vi "GetAlarms.vi"(0 "reference in":refnum<class "Stand.lvclass">, 11 "error in (no error)":errorcluster) -> (4 "reference out":refnum<class "Stand.lvclass">, 6 "Alarm":bool, 8 "Warning":bool, 15 "error out":errorcluster)   [LabVIEW 2019, in "Stand.lvclass"]
uses:
  Stand.lvclass
  Stand.lvclass/Stand.ctl
  PM_Group_class/PM_Group.lvclass
  C:/Users/ANENKOV_V1/Desktop/src/Proccess_class/Proccess.lvclass
  NeedleValve_class/NeedleValve.lvclass
  AI_class/AI.lvclass
  DI_class/DI.lvclass
  Valve_2DO_2DI_class/Valve_2DO_2DI.lvclass
  DA_class/DA.lvclass
  Proccess_class/Proccess.lvclass
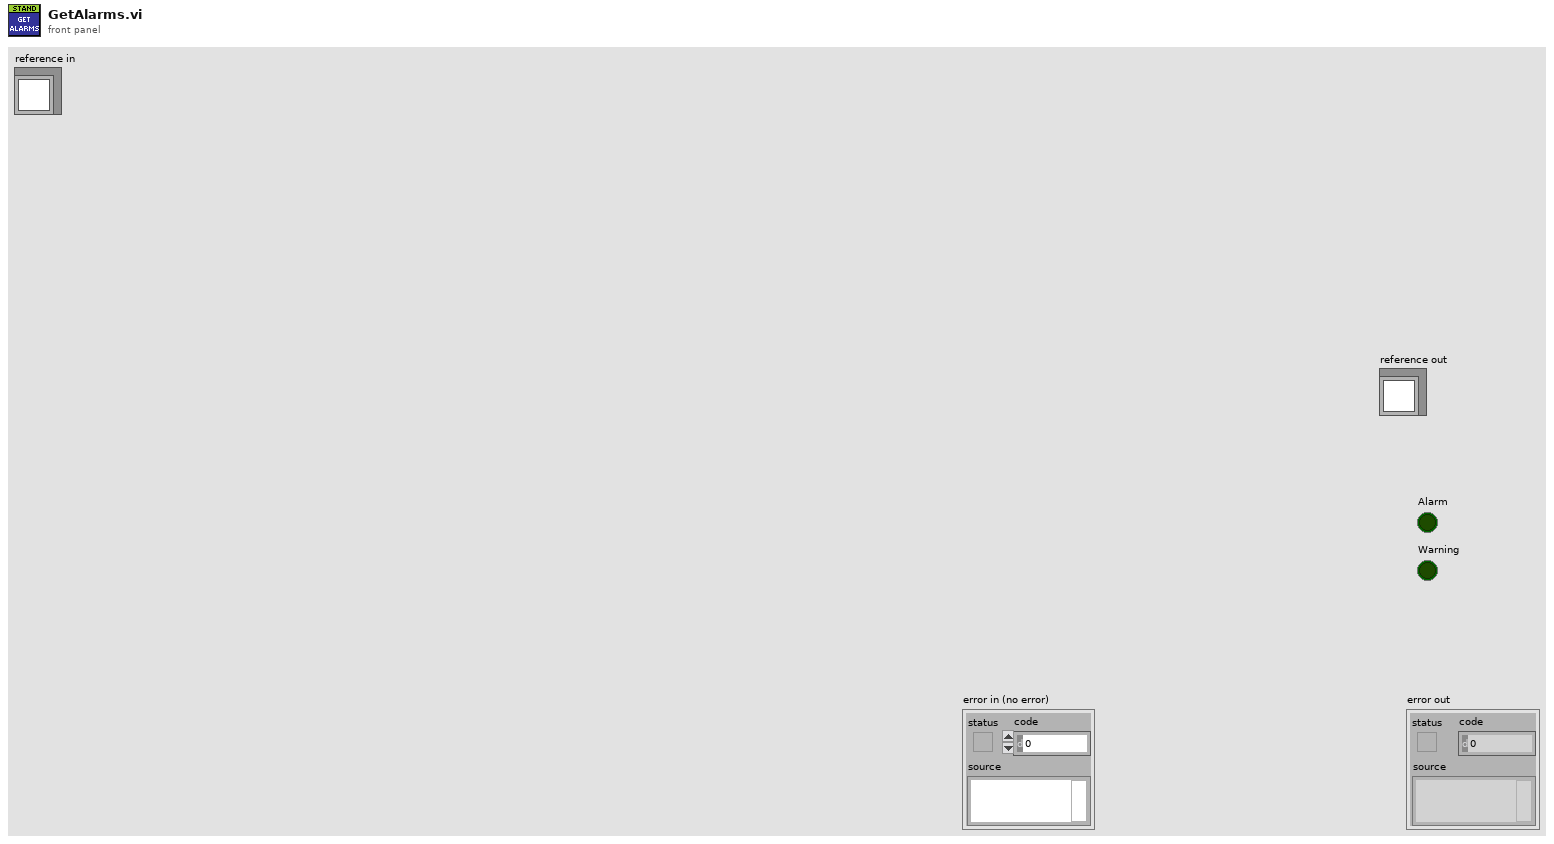
[diagram p1: front panel]
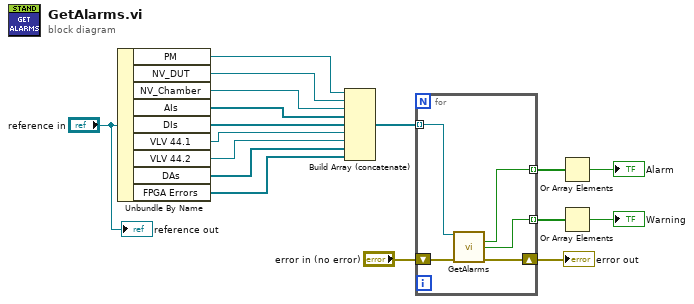
[diagram p0: block diagram]
diagram:
  n1 = Unbundle By Name("reference in") -> ("PM"=w9:refnum<class "PM_Group.lvclass">, "NV_DUT"=w8:refnum<class "NeedleValve.lvclass">, "NV_Chamber"=w7:refnum<class "NeedleValve.lvclass">, "AIs"=w6:refnum<class "AI.lvclass">[], "DIs"=w5:refnum<class "DI.lvclass">[], "VLV 44.1"=w4:refnum<class "Valve_2DO_2DI.lvclass">, "VLV 44.2"=w3:refnum<class "Valve_2DO_2DI.lvclass">, "DAs"=w2:refnum<class "DA.lvclass">[], "FPGA Errors"=w1:refnum<class "DA.lvclass">[])
  n2 = Build Array (concatenate)(w9, w8, w7, w6, w5, w4, w3, w2, w1) -> (w16:refnum<class "Proccess.lvclass">[])
  n3 = for {
    tunnel: w16 -> [w22] mode=indexing
    tunnel: [w21] -> w15 mode=indexing
    tunnel: [w20] -> w14 mode=indexing
    shift-right: [w19] -> w12
    shift-left: "error in (no error)" -> [w18]
    n4 = call-dynamic "GetAlarms.vi"("Proccess in"=w22, "error in (no error)"=w18) -> ("Alarm"=w21:bool, "Warning"=w20:bool, "error out"=w19:errorcluster)  [unwired: 10 in, 1 out]
  }
  "error out" <- w12
  n5 = Or Array Elements(Boolean array=w15) -> (logical OR=→"Alarm":bool)
  n6 = Or Array Elements(Boolean array=w14) -> (logical OR=→"Warning":bool)
  "reference out" <- "reference in"
